vi "Set Pre-Execution Icons.vi"(8 "error in (no error)":errorcluster, 10 "Test Suite":refnum<class "LUnit Test Suite.lvclass">, 11 "Test Tree In":refnum<class "Test Result Tree.lvclass">) -> (0 "error out":errorcluster, 3 "Test Tree Out":refnum<class "Test Result Tree.lvclass">)   [LabVIEW 2020, in "Test Result Tree.lvclass"]
uses:
  Framework/Helper Classes/Test Result Tree/Test Result Tree.lvclass
  C:/Git/astemes-lunit/source/Rewrite Project/Test Tree/Test Tree.lvclass
  Framework/Test Suite/LUnit Test Suite.lvclass
  Test Tree.lvclass/Test Tree.ctl
  Framework/Test Suite/LUnit Test Suite.lvclass/LUnit Test Suite.ctl
  Framework/Test Case/LUnit Test Case.lvclass/LUnit Test Case.ctl
  Framework/Test Case/LUnit Test Case.lvclass
  Test Tree.lvclass
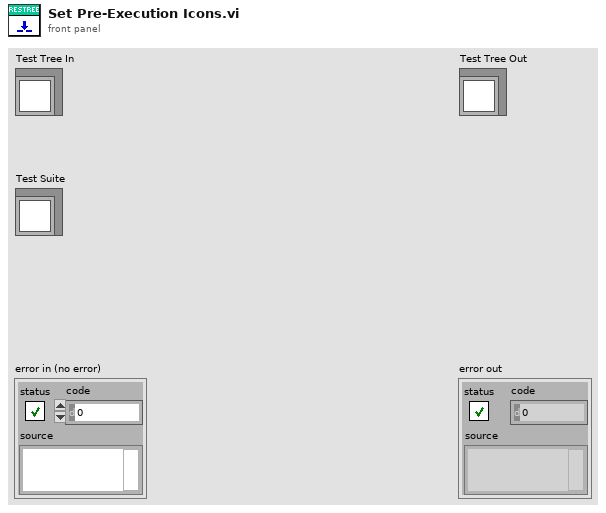
[diagram p1: front panel]
types:
  T1 = map{string, cluster{"Left Cell String":string, "Child Text":string[], "Item Indent":i32, "Child Only?":bool, "Glyph Index":i32}}
  T2 = cluster{"Left Cell String":string, "Child Text":string[], "Item Indent":i32, "Child Only?":bool, "Glyph Index":i32}
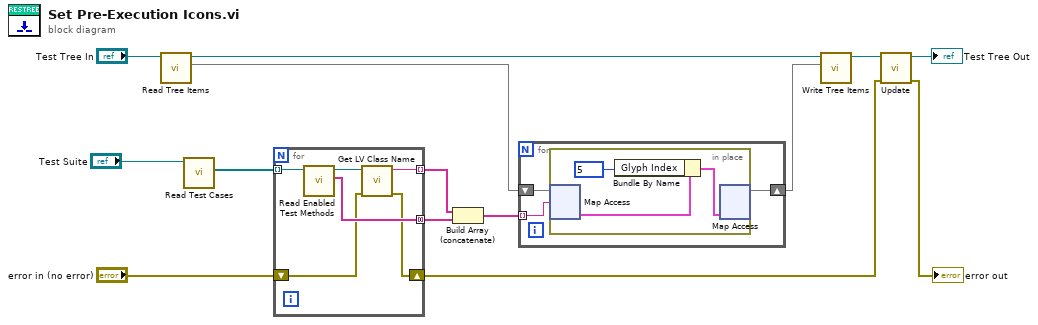
[diagram p0: block diagram]
diagram:
  n1 = call "Read Tree Items.vi"("Test Tree In"="Test Tree In") -> ("Tree Items"=w2:T1, "Test Tree Out"=w3:refnum<class "Test Result Tree.lvclass">)  [unwired: 9 in]
  n2 = call "Read Test Cases.vi"("Test Suite In"="Test Suite") -> ("Test Cases"=w13:refnum<class "LUnit Test Case.lvclass">[])  [unwired: 9 in, 1 out]
  n3 = for {
    tunnel: w13 -> [w20] mode=indexing
    shift-right: [w18] -> w10
    shift-left: "error in (no error)" -> [w15]
    tunnel: [w19] -> w12 mode=concatenating
    tunnel: [w16] -> w8 mode=indexing
    n4 = call "Read Enabled Test Methods.vi"("LUnit Test Case In"=w20) -> ("Names"=w19:string[], "LUnit Test Case Out"=w17:refnum<class "LUnit Test Case.lvclass">)  [unwired: 8 in, 1 out]
    n5 = call <vilib>:"Get LV Class Name.vi"("error in (no error)"=w15, "object"=w17) -> ("error out"=w18:errorcluster, "class name"=w16:string)  [unwired: 8 in]
  }
  n6 = Build Array (concatenate)(w8, w12) -> (w7:string[])
  n7 = for {
    tunnel: w7 -> [w22] mode=indexing
    shift-right: [w21] -> w6
    shift-left: w2 -> [w23]
    n8 = in-place {
      n9 = in-place-map #1(w23, w22) -> (w26:T2)  [unwired: 1 in, 1 out]
      n10 = Bundle By Name(cluster=w26, "Glyph Index"=5 ("Listbox Symbol Ring Constant")) -> (w25:T2)
      n11 = in-place-map #1(w25) -> (w21:T1)  [unwired: 1 in, 2 out]
    }
  }
  n12 = call "Write Tree Items.vi"("Tree Items"=w6, "Test Tree In"=w3) -> ("Test Tree Out"=w5:refnum<class "Test Result Tree.lvclass">)  [unwired: 9 in]
  n13 = call "Update.vi"("error in (no error)"=w10, "Test Tree In"=w5) -> ("error out"=→"error out":errorcluster, "Test Tree Out"=→"Test Tree Out":refnum<class "Test Result Tree.lvclass">)  [unwired: 8 in]
